vi "LineDetection-Circle.vi"() -> ()   [LabVIEW 2014]
doc: "This example shows how to use the Edge Tool in NI Vision. The Edge Tool finds edges (or sharp transitions in the pixels values) along a given line or ROI profile. The Edge Tool is a precursor function to many of the gauging and inspection tasks. For example, the location of the edges found along a line profile across an object can interpreted as the boundaries of the object whose dimensions have to be measured for a gauging application or the presence of a crack in the surface of an object for an inspection application."
uses:
  <vilib>/vision/Measure.llb/Edge Options.ctl
  <vilib>/vision/Measure.llb/Edge Polarity.ctl
  <vilib>/vision/NI_Vision_Development_Module.lvlib
panel:
  in  "Options":T3={"Search  Direction"=0, "Edge Options"={"Edge Polarity"=0, "Kernel Size"=3, "Width"=3, "Minimum Edge Strength"=10.0, "Interpolation Type"=enum."Bilinear Fixed", "Data Processing Method"=enum."Average"}, "Show Search Area"=FALSE, "Show Search Lines"=FALSE, "Show Edges Found"=FALSE, "Show Result"=TRUE, "Search Area Color"=65280, "Search Lines Color"=255, "Edge Locations Color"=16776960, "Result Color"=16711680, "Overlay Group Name"=""} {"Search  Direction" items=["Outside to Inside", "Inside to Outside"]; "Edge Options"."Edge Polarity" items=["All Edges", "Rising Edges", "Falling Edges"]; "Edge Options"."Minimum Edge Strength" format="%.2f"; "Edge Options"."Width" step=2; "Edge Options"."Kernel Size" step=2}
  in  "Circle Fit Options":T4={"Process"=enum."Get First Edge", "Step Size"=30.0, "Max Pixel Radius"=3}
  out "Image":T5(plugin-control)
  in  "Stop":bool
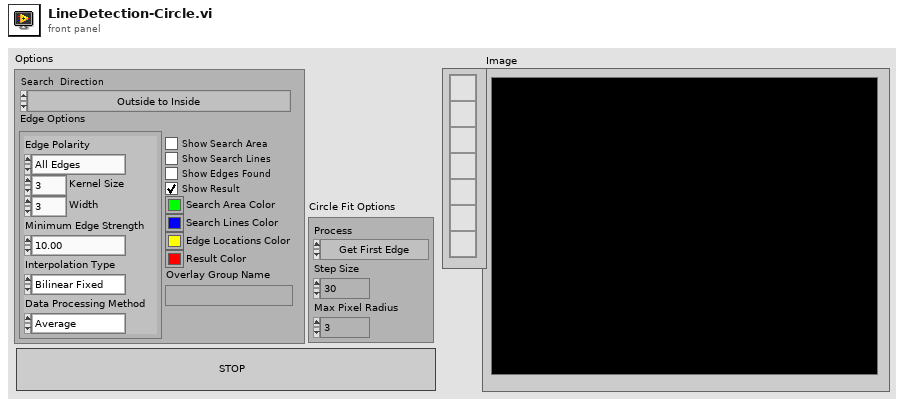
[diagram p1: front panel]
types:
  T1 = typedef "Edge Options.ctl" = cluster{"Edge Polarity":T2, "Kernel Size":u32, "Width":u32, "Minimum Edge Strength":sgl, "Interpolation Type":enum32{"Zero Order", "Bilinear", "Quadratic", "Cubic", "Bilinear Fixed"}, "Data Processing Method":enum32{"Average", "Median"}}
  T2 = typedef "Edge Polarity.ctl" = u32
  T3 = cluster{"Search  Direction":u32, "Edge Options":T1, "Show Search Area":bool, "Show Search Lines":bool, "Show Edges Found":bool, "Show Result":bool, "Search Area Color":u32, "Search Lines Color":u32, "Edge Locations Color":u32, "Result Color":u32, "Overlay Group Name":string}
  T4 = cluster{"Process":enum16{"Get First Edge", "Get First + Last Edge", "Get All Edges", "Get Best Edge"}, "Step Size":dbl, "Max Pixel Radius":i32}
  T5 = typedef "IMAQ Image.ctl" = refnum<image>
  T6 = typedef "IMAQ Circle" = cluster{"Center X":i32, "Center Y":i32, "Inner Radius":i32, "Outer Radius":i32, "Start Angle":dbl, "End Angle":dbl}
  T7 = typedef "ROI Descriptor" = cluster{"Global Rectangle":i32[], "Contours":cluster{"ID":enum32{"External", "Internal"}, "Type":u32, "Coordinates":i32[]}[]}
  T8 = cluster{"Options":cluster{"Search  Direction":u32, "Edge Options":T1, "Show Search Area":bool, "Show Search Lines":bool, "Show Edges Found":bool, "Show Result":bool, "Search Area Color":u32, "Search Lines Color":u32, "Edge Locations Color":u32, "Result Color":u32, "Overlay Group Name":string}, "Circle Fit Options":cluster{"Process":enum16{"Get First Edge", "Get First + Last Edge", "Get All Edges", "Get Best Edge"}, "Step Size":dbl, "Max Pixel Radius":i32}}
  T9 = cluster{"Global Rectangle":i32[], "Contours":cluster{"Contour Type":u32, "ROI Type":u32, "Points":i32[]}[]}
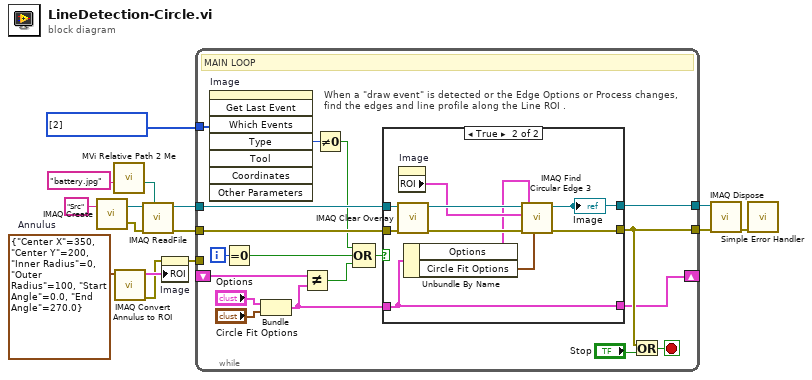
[diagram p0: block diagram]
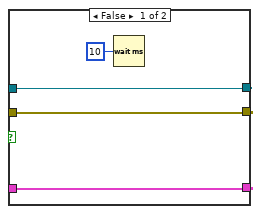
[diagram p2: hidden frame]
diagram:
  w1 = T6 {"Center X"=350, "Center Y"=200, "Inner Radius"=0, "Outer Radius"=100, "Start Angle"=0.0, "End Angle"=270.0}  # Annulus
  w7 = i32[] [2] items=["No  event", "Click event", "Draw event", "Move event", "Size event", "Scroll event", "Activate event", "Close event", "Double click event"] ("Events list (all)")
  n1 = call "IMAQ Create"("Image Name"="Src") -> ("New Image"=w14:T5, "error out"=w13:errorcluster)  [unwired: 4 in]
  n2 = call "MVi Relative Path 2 Me.vi"("Relative Path"="battery.jpg" ("name or relative path")) -> ("Appended Dir"=w5:path)  [unwired: 5 in, 1 out]
  n3 = call "IMAQ Convert Annulus to ROI"("Annulus"=w1) -> ("error out"=w3:errorcluster, "ROI Descriptor"=w4:T7)  [unwired: 8 in]
  n4 = call "IMAQ ReadFile"("File Path"=w5, "error in (no error)"=w13, "Image"=w14) -> ("error out"=w8:errorcluster, "Image Out"=w9:T5)  [unwired: 4 in, 3 out]
  n5 = property on="Image" class="ImageControl"(error in=w3, "ROI"=w4) -> (error out=w2:errorcluster)  [unwired: 1 in, 1 out]
  n6 = while "MAIN LOOP" {
    tunnel: w9 -> [w32]
    tunnel: w8 -> [w33]
    tunnel: [w28] -> w12
    tunnel: [w29] -> w11
    tunnel: w7 -> [w27]
    shift-right: [w22] -> _
    shift-left: _ -> [w19]
    tunnel: w2 -> [_]
    i -> [w25]
    stop <- w30 stop-if-true
    # "When a \"draw event\" is detected or the Edge Options or Process changes, find the edges and line profile along the Line ROI ."
    # "MAIN LOOP"
    n7 = invoke on="Image" class="ImageControl" method="Get Last Event"("Which Events"=w27) -> ("Type"=w26:i32)  [unwired: 7 in, 7 out]
    n8 = Equal To 0?(x=w25) -> (x = 0?=w21:bool)
    n9 = Bundle("Options"="Options", "Circle Fit Options"="Circle Fit Options") -> (w20:T8)  [unwired: 1 in]
    n10 = Not Equal?(x=w19, y=w20) -> (x != y?=w18:bool)
    n11 = Not Equal To 0?(x=w26) -> (x != 0?=w24:bool)
    n12 = Compound Arithmetic op=OR(w24, w21, w18) -> (w23:bool)
    n13 = case shown="True" w23 {
      tunnel: w33 -> [w36 w47]
      tunnel: w32 -> [w37 w46]
      tunnel: [w37 w40] -> w29
      tunnel: [w36 w41] -> w28
      tunnel: [w34 w45] -> w22
      tunnel: w20 -> [w34 w45]
      frame False {
        n14 = Wait (ms)(milliseconds to wait=u32 10) -> ()  [unwired: 1 out]
      }
      frame True {
        n15 = call "IMAQ Clear Overlay"("error in (no error)"=w47, "Image"=w46) -> ("error out"=w44:errorcluster, "Image Out"=w43:T5)  [unwired: 8 in]
        n16 = property on="Image" class="ImageControl"() -> ("ROI"=w42:T9)  [unwired: 2 in, 2 out]
        n17 = Unbundle By Name(w45) -> ("Options"=w39:T3, "Circle Fit Options"=w38:T4)
        n18 = call "IMAQ Find Circular Edge 3"("Circle Fit Options"=w38, "Options"=w39, "error in (no error)"=w44, "ROI Descriptor"=w42, "Image"=w43) -> ("error out"=w41:errorcluster, "Image Out"=w40:T5)  [unwired: 2 in, 3 out]
        "Image" <- w40
      }
    }
    n19 = Or(x=w28, y="Stop") -> (x .or. y?=w30:bool)
  }
  n20 = call "IMAQ Dispose"("Image"=w11, "error in (no error)"=w12) -> ("error out"=w10:errorcluster)  [unwired: 4 in]
  n21 = call <vilib>:"Simple Error Handler.vi"("error in (no error)"=w10) -> ()  [unwired: 4 in, 5 out]
